vi "Add to Array.vi"(0 "Database Entry in":refnum<class "Database Entry.lvclass">, 1 "Operator":string, 2 "Temp and RelHumidity":T1, 5 "Position Index":dbl, 7 "Module type":string, 9 "Module?":bool, 11 "error in (no error)":errorcluster, 12 "Adhesive":string, 13 "ROC version":string) -> (4 "Database Entry out":refnum<class "Database Entry.lvclass">, 8 "Position cancelled?":bool, 15 "error out":errorcluster)   [LabVIEW 2021, in "Database Entry.lvclass"]
uses:
  Database Entry.lvclass
  Components/Stack/Stack.lvclass
  Database Entry.lvclass/Database Entry.ctl
panel:
  out "Array":dbl[](array[numeric])
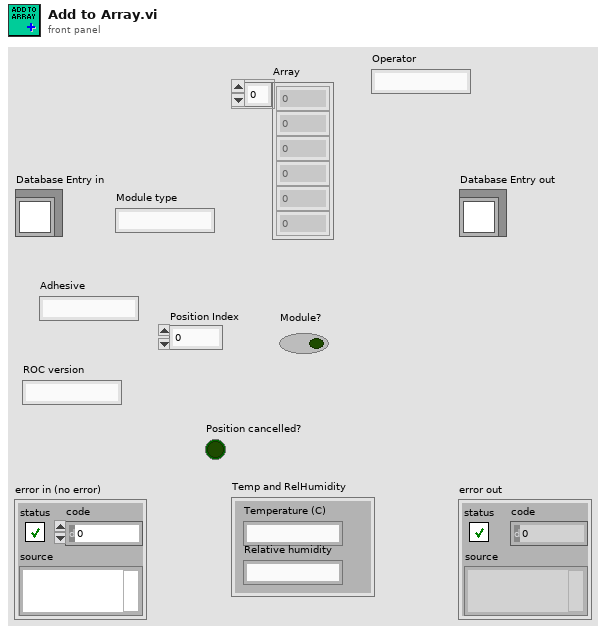
[diagram p1: front panel]
types:
  T1 = cluster{"Temperature (C)":string, "Relative humidity":string}
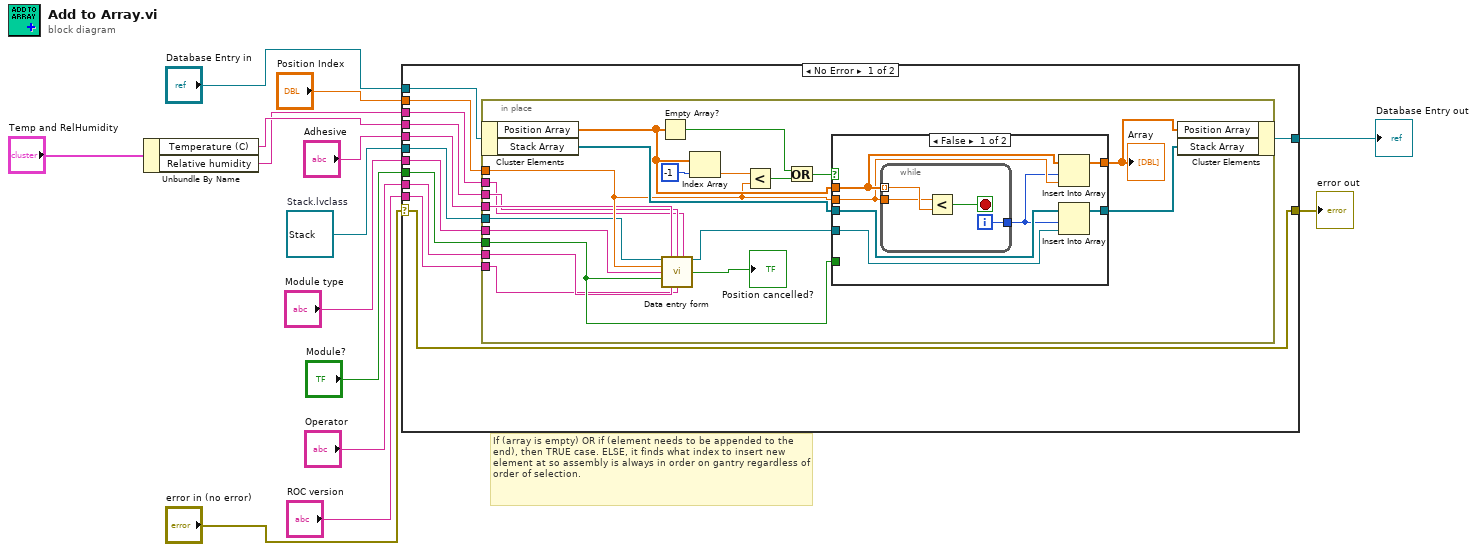
[diagram p0: block diagram]
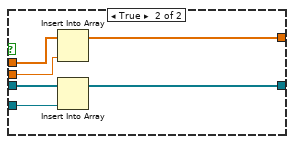
[diagram p2: hidden frame]
diagram:
  w9 = refnum<class "Stack.lvclass"> refnum  # Stack.lvclass
  # "If (array is empty) OR if (element needs to be appended to the end), then TRUE case. ELSE, it finds what index to insert new element at so assembly is always in order on gantry regardless of order of selection."
  n1 = Unbundle By Name("Temp and RelHumidity") -> ("Temperature (C)"=w2:string, "Relative humidity"=w1:string)
  n2 = case shown="No Error" "error in (no error)" {
    selector: "error in (no error)" -> [w26 w65]
    tunnel: [w26 w65] -> w13
    tunnel: [w23 w64] -> w11
    tunnel: "Database Entry in" -> [w24 w64]
    tunnel: w9 -> [w25 _]
    tunnel: "Position Index" -> [w22 _]
    tunnel: "Module?" -> [w21 _]
    tunnel: "Operator" -> [w20 _]
    tunnel: "Module type" -> [w19 _]
    tunnel: "Adhesive" -> [w18 _]
    tunnel: "ROC version" -> [w17 _]
    tunnel: w2 -> [w16 _]
    tunnel: w1 -> [w15 _]
    frame No Error {
      n3 = in-place {
        in-place-border: w25 -> [w35]
        in-place-border: w22 -> [w37]
        in-place-border: w21 -> [w36]
        in-place-border: w20 -> [w34]
        in-place-border: w19 -> [w33]
        in-place-border: w18 -> [w32]
        in-place-border: w17 -> [w31]
        in-place-border: w16 -> [w28]
        in-place-border: w15 -> [w27]
        n4 = in-place-cluster #1(w24) -> ("Position Array"=w44:dbl[], "Stack Array"=w46:refnum<class "Stack.lvclass">[])
        n5 = Empty Array?(array=w44) -> (empty?=w41:bool)
        n6 = call "Data entry form.vi"("Stack in"=w35, "Adhesive type"=w32, "Temperature (C)"=w28, "Relative humidity"=w27, "Position"=w37, "Module Type"=w33, "Module?"=w36, "Operator"=w34, "ROC version"=w31) -> ("Stack out"=w38:refnum<class "Stack.lvclass">, "Cancelled?"=→"Position cancelled?":bool)  [unwired: 4 in, 1 out]
        n7 = Index Array(array=w44, index=-1) -> (element=w42:dbl)
        n8 = Less?(x=w42, y=w37) -> (x < y?=w40:bool)
        n9 = Or(x=w41, y=w40) -> (x .or. y?=w39:bool)
        n10 = case shown="False" w39 {
          tunnel: w46 -> [w51 w61]
          tunnel: [w52 w59] -> w30
          tunnel: [w53 w63] -> w45
          tunnel: w36 -> [_ _]
          tunnel: w37 -> [w48 w60]
          tunnel: w44 -> [w49 w62]
          tunnel: w38 -> [w50 w58]
          frame False {
            n11 = while {
              tunnel: w49 -> [w57] mode=indexing
              tunnel: w48 -> [w56]
              tunnel: [w54] -> w47
              i -> [w54]
              stop <- w55 stop-if-true
              n12 = Less?(x=w56, y=w57) -> (x < y?=w55:bool)
            }
            n13 = Insert Into Array(array=w49, index=w47, new element=w48) -> (w53:dbl[])
            n14 = Insert Into Array(array=w51, index=w47, new element=w50) -> (w52:refnum<class "Stack.lvclass">[])
          }
          frame True {
            n15 = Insert Into Array(array=w62, new element=w60) -> (w63:dbl[])  [unwired: 1 in]
            n16 = Insert Into Array(array=w61, new element=w58) -> (w59:refnum<class "Stack.lvclass">[])  [unwired: 1 in]
          }
        }
        "Array" <- w45
        n17 = in-place-cluster #1("Position Array"=w45, "Stack Array"=w30) -> (w23:refnum<class "Database Entry.lvclass">)
      }
    }
    frame Error {
    }
  }
  "error out" <- w13
  "Database Entry out" <- w11
